vi "FTW-CodeGen-GetErrors.vi"(5 "FTW XNode State":T1 {"TotalCodeGens" format="CodeGens:   %04d"; "TotalAdaptToInputs" format="AdaptTerms: %04d"; "FinishedCodegen" format="%_3psec"; "ElapsedTilCodegen" format="%_3psec"; "AdaptToInputsBegin" format="%.3fmsec\n%<%D:%H:%M:%S%3u>t"}, 9 "Generate Strings?":bool) -> (6 "Errors":T6(array[cluster]), 10 "Errors Present?":bool)   [LabVIEW 2015]
uses:
  FTW-CodeGen-XNodeCommonState.ctl
  FTW-CodeGen-XNodeAdaptiveTerminal.ctl
  FTW-CodeGen-XNodeAdaptiveTerminal-Controller.ctl
  src/reflection/FTW-Reflection-Types.ctl
  FTW-CodeGen-XNodeAdaptiveTerminal-ControllerBehavior.ctl
panel:
  # "Inputs"
  # "Outputs"
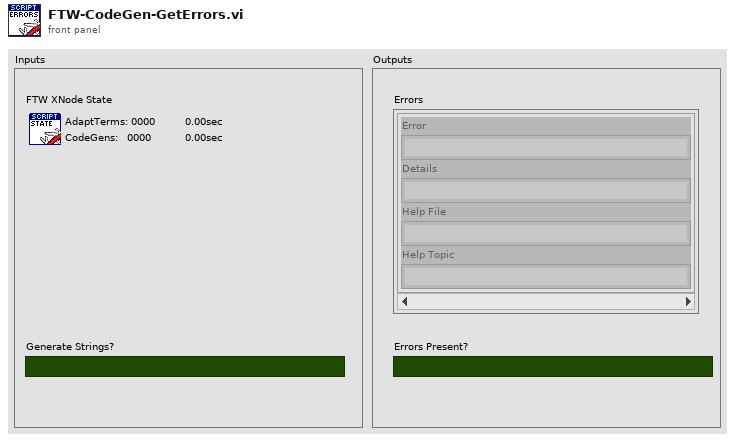
[diagram p1: front panel]
types:
  T1 = typedef "FTW-CodeGen-XNodeCommonState.ctl" = cluster{"Terms":cluster{"Name":string, "Id":string, "Type":variant, "Bounds":cluster{"Left":i32, "Top":i32, "Right":i32, "Bottom":i32}, "Input?":bool, "Required?":bool, "Recommended?":bool, "Adaptive?":bool, "Hidden?":bool, "Direction":enum32{"Auto", "Up", "Down", "Left", "Right", "Center"}, "Break Wire?":bool, "English Name":string}[], "AdaptiveTerms":T2[], "AdaptiveTerminalsOK":bool, "ForceCodeRegeneration?":bool, "LastGeneration":timestamp, "CodeGenError":errorcluster, "AdaptToInputsBegin":dbl, "ElapsedTilCodegen":dbl, "FinishedCodegen":dbl, "TotalAdaptToInputs":i32, "TotalCodeGens":i32}
  T2 = typedef "FTW-CodeGen-XNodeAdaptiveTerminal.ctl" = cluster{"Config":T3, "ID":string, "ParentIndex":i32, "Wired?":bool, "WiredTypeAllowed?":bool, "LastValidWireName":string, "LastValidWireType":T4, "Followers":i32[]}
  T3 = typedef "FTW-CodeGen-XNodeAdaptiveTerminal-Controller.ctl" = cluster{"AllowedTypes":T4[], "UnconstrainedTypeBehavior":T5, "DefaultType":variant}
  T4 = typedef "FTW-Reflection-Types.ctl" = enum16{"Unknown", "Void", "Array", "Cluster", "LVObject", "Boolean", "I8", "I16", "I32", "I64", "U8", "U16", "U32", "U64", "SGL", "DBL", "EXT", "CSG", "CDB", "CXT", "FXP", "EnumU8", "EnumU16", "EnumU32", "EnumU64", "SGLwithUnit", "DBLwithUnit", "EXTwithUnit", "CSGwithUnit", "CDBwithUnit", "CXTwithUnit", "String", "Path", "Picture", "Tag", "LVVariant", "Timestamp", "WaveformI8", "WaveformI16", "WaveformI32", "WaveformI64", "WaveformU8", "WaveformU16", "WaveformU32", "WaveformU64", "WaveformSGL", "WaveformDBL", "WaveformEXT", "WaveformCSG", "WaveformCDB", "WaveformCXT", "WaveformDigital", "WaveformUnknownType", "DigitalData", "DynamicData", "ExternalData", "FileByteStream", "TDMStream", "dotNET", "ActiveX", "VIServerReference", "VIReference", "ApplicationInstance", "Menu", "ConnectionDataSocket", "ConnectionVISA", "ConnectionBluetooth", "ConnectionIrDA", "ConnectionTCP", "ConnectionUDP", "ConnectionHTTPClient", "ConnectionFTP", "Occurrence", "Notifier", "Queue", "Rendezvous", "Semaphore", "RTFIFO", "EventPublisher", "EventRegistration", "EventCallback", "DataValueReference", "GenericClass", "GenericClassTag", "GenericClassDeepCopy", "GenericClassFlattened", "GenericClassTagFlattened", "GenericReferenceType", "WindowsRegistry", "OverloadedDatalogRef", "ReferenceUnknownType", "ByteArray", "ConPaneInterface", "FTWObject"}
  T5 = typedef "FTW-CodeGen-XNodeAdaptiveTerminal-ControllerBehavior.ctl" = enum16{"UseDefaultType", "StickyToLastValidType"}
  T6 = cluster{"Error":string, "Details":string, "Help File":string, "Help Topic":string}[]
  T7 = cluster{"Error":string, "Details":string, "Help File":string, "Help Topic":string}
  T8 = typedef "FTW-ERR-ExceptionType.ctl" = enum16{"OK", "Info", "Warning", "Error"}
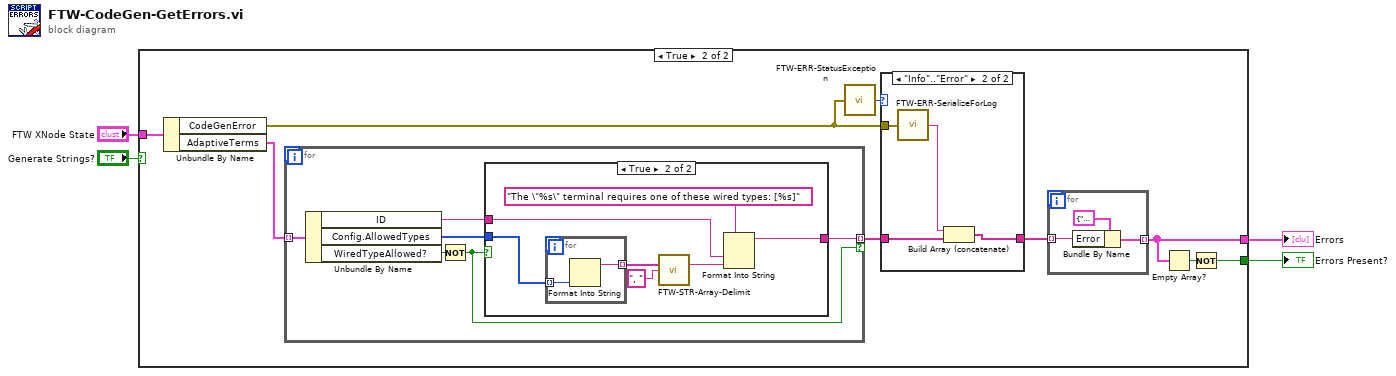
[diagram p0: block diagram]
diagram:
  n1 = case shown="True" "Generate Strings?" {
    tunnel: "FTW XNode State" -> [_ w13]
    tunnel: [_ w12] -> w3
    tunnel: [_ w10] -> w2
    frame False {
    }
    frame True {
      n2 = Unbundle By Name(w13) -> ("CodeGenError"=w7:errorcluster, "AdaptiveTerms"=w9:T2[])
      n3 = for {
        tunnel: w9 -> [w27] mode=indexing
        tunnel: [w25] -> w6 mode=indexing if=w23
        n4 = Unbundle By Name(w27) -> ("ID"=w26:string, "Config.AllowedTypes"=w24:T4[], "WiredTypeAllowed?"=w22:bool)
        n5 = Not(x=w22) -> (.not. x?=w23:bool)
        n6 = case shown="True" w23 {
          tunnel: w26 -> [_ w28]
          tunnel: w24 -> [_ w34]
          tunnel: [_ w29] -> w25
          frame False {
          }
          frame True {
            n7 = for {
              tunnel: w34 -> [w36] mode=indexing
              tunnel: [w35] -> w33 mode=indexing
              n8 = Format Into String(w36) -> (resulting string=w35:string)  [unwired: 3 in, 1 out]
            }
            n9 = call "FTW-STR-Array-Delimit.vi"("Array of Strings"=w33, "Delimiter"=", ") -> ("Delimited String"=w30:string)  [unwired: 13 in]
            n10 = Format Into String(format string="The \"%s\" terminal requires one of these wired types: [%s]" ("string"), w28, w30) -> (resulting string=w29:string)  [unwired: 2 in, 1 out]
          }
        }
      }
      n11 = call "FTW-ERR-StatusException.vi"("error to check"=w7) -> ("Exception"=w8:T8)
      n12 = case shown="\"Info\"..\"Error\"" w8 {
        tunnel: w7 -> [_ w18]
        tunnel: w6 -> [w14 w16]
        tunnel: [w14 w15] -> w5
        frame "OK" {
        }
        frame "Info".."Error" {
          n13 = call "FTW-ERR-SerializeForLog.vi"("error in"=w18) -> ("Serialized Error"=w17:string)
          n14 = Build Array (concatenate)(w17, w16) -> (w15:string[])
        }
      }
      n15 = for {
        tunnel: w5 -> [w20] mode=indexing
        tunnel: [w19] -> w12 mode=indexing
        n16 = Bundle By Name(cluster=T7 {"Error"="", "Details"="", "Help File"="", "Help Topic"=""} ("Error"), "Error"=w20) -> (w19:T7)
      }
      n17 = Empty Array?(array=w12) -> (empty?=w11:bool)
      n18 = Not(x=w11) -> (.not. x?=w10:bool)
    }
  }
  "Errors" <- w3
  "Errors Present?" <- w2
